vi "Main.vi"() -> ()   [LabVIEW 2023]
panel:
  out "Celsius":dbl(slide) scale=0.0..100.0
  out "Fahrenheit":dbl(slide) scale=0.0..100.0
  in  "Exit":bool
  in  "Add Sensor":bool
  in  "Listbox":i32(listbox)
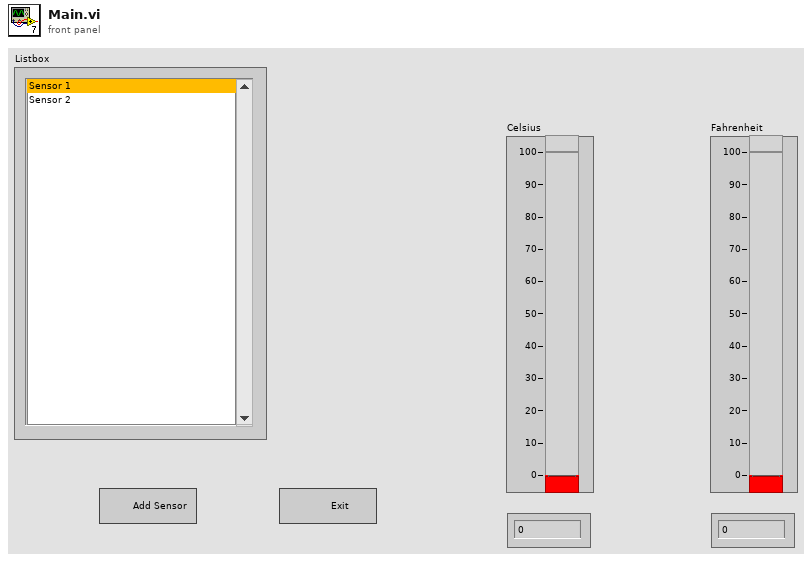
[diagram p1: front panel]
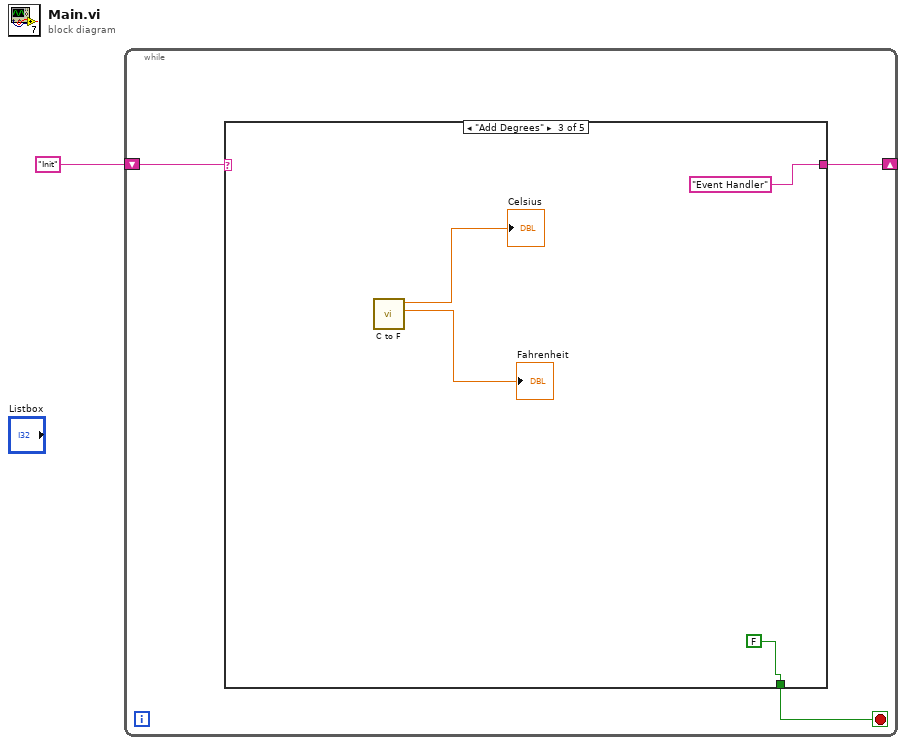
[diagram p0: block diagram]
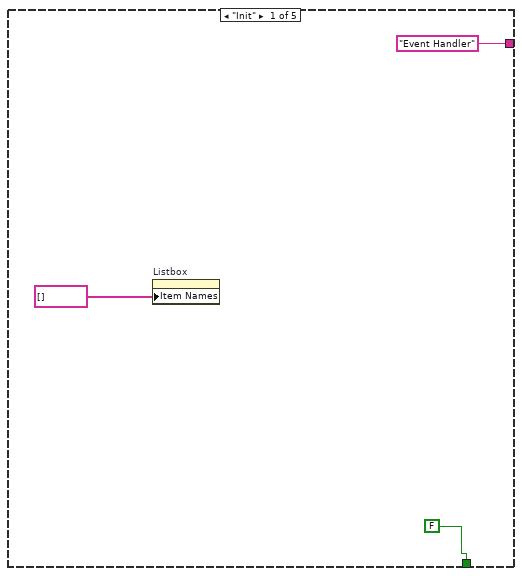
[diagram p2: hidden frame]
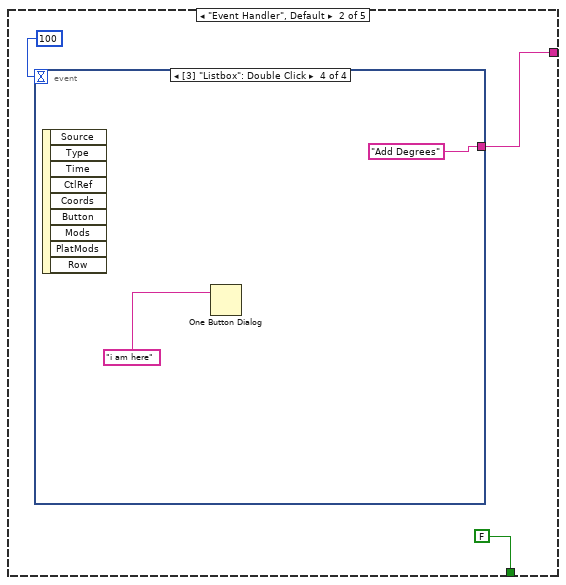
[diagram p3: hidden frame]
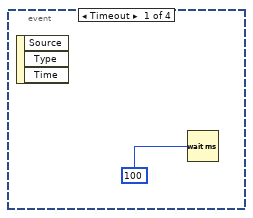
[diagram p4: hidden frame]
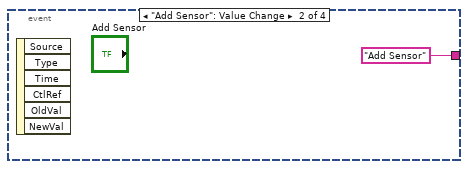
[diagram p5: hidden frame]
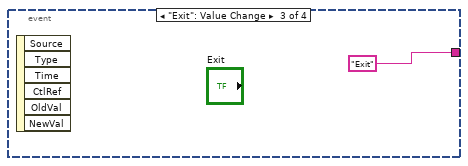
[diagram p6: hidden frame]
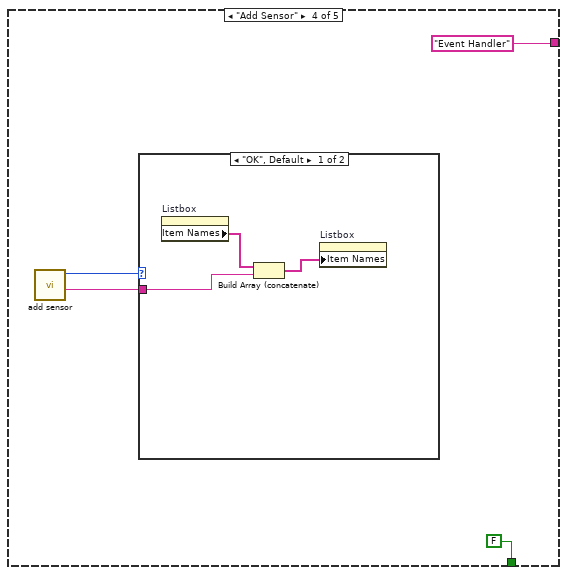
[diagram p7: hidden frame]
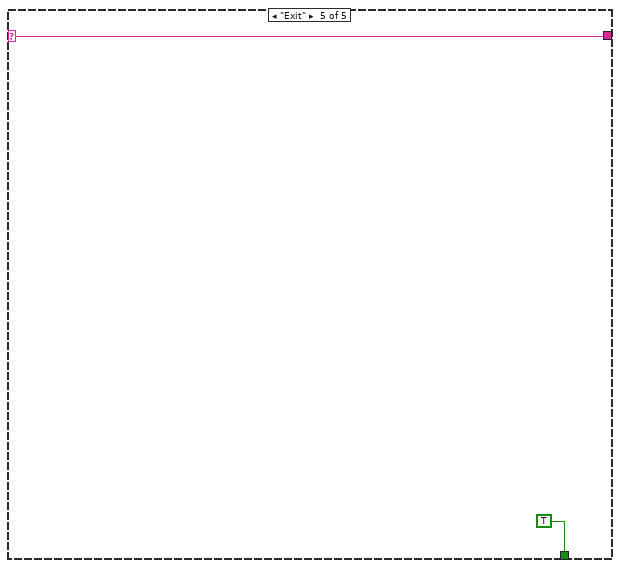
[diagram p9: hidden frame]
diagram:
  n1 = while {
    shift-right: [w3] -> _
    shift-left: "Init" -> [w4]
    stop <- w2 stop-if-true
    n2 = case shown="\"Add Degrees\"" w4 {
      selector: w4 -> [_ _ _ _ w27]
      tunnel: ["Event Handler" w9 "Event Handler" "Event Handler" w27] -> w3
      tunnel: [FALSE FALSE FALSE FALSE TRUE] -> w2
      frame "Init" {
        n3 = property on="Listbox" class="LstBox (strict)"("Item Names"=string[] []) -> ()  [unwired: 2 in, 2 out]
      }
      frame "Event Handler", Default {
        n4 = event shown="[3] \"Listbox\": Double Click" {
          selector: _ -> [_ _ _ _]
          dyn-events: _ -> [_ _ _ _]
          timeout: 100 -> [_ _ _ _]
          tunnel: [_ "Add Sensor" "Exit" "Add Degrees"] -> w9
          event Timeout {
            n5 = event-data() -> ()  [unwired: 1 in, 3 out]
            n6 = Wait (ms)(milliseconds to wait=u32 100) -> ()  [unwired: 1 out]
          }
          event "Add Sensor": Value Change {
            n7 = event-data() -> ()  [unwired: 1 in, 6 out]
          }
          event "Exit": Value Change {
            n8 = event-data() -> ()  [unwired: 1 in, 6 out]
          }
          event "Listbox": Double Click {
            n9 = event-data() -> ()  [unwired: 1 in, 9 out]
            n10 = One Button Dialog(message="i am here") -> ()  [unwired: 1 in, 1 out]
          }
        }
      }
      frame "Add Degrees" {
        n11 = call "C to F.vi"() -> ("x+y"=→"Fahrenheit":dbl, "number"=→"Celsius":dbl)  [unwired: 9 in, 1 out]
      }
      frame "Add Sensor" {
        n12 = call "add sensor.vi"() -> ("new sensor output"=w22:string, "Enum"=w23:enum16{"OK", "Cancel"})  [unwired: 9 in, 1 out]
        n13 = case shown="\"OK\", Default" w23 {
          tunnel: w22 -> [w25 _]
          frame "OK", Default {
            n14 = property on="Listbox" class="LstBox (strict)"() -> ("Item Names"=w26:string[])  [unwired: 2 in, 2 out]
            n15 = Build Array (concatenate)(w26, w25) -> (w24:string[])
            n16 = property on="Listbox" class="LstBox (strict)"("Item Names"=w24) -> ()  [unwired: 2 in, 2 out]
          }
          frame "Cancel" {
          }
        }
      }
      frame "Exit" {
      }
    }
  }
